vi "Handle Payload.vi"(8 "error in (no error)":errorcluster, 10 "Incoming Packets":u8[](array[numeric]) format="%08b", 11 "ControlPacket in":refnum<class "ControlPacket.lvclass">) -> (0 "error out":errorcluster, 1 "Payload Complete?":bool=TRUE, 2 "Remaining Packets":u8[](array[numeric]) format="%08b", 3 "ControlPacket out":refnum<class "ControlPacket.lvclass">)   [LabVIEW 2013, in "ControlPacket.lvclass"]
uses:
  ControlPacket.lvclass
  ControlPacket.lvclass/ControlPacket.ctl
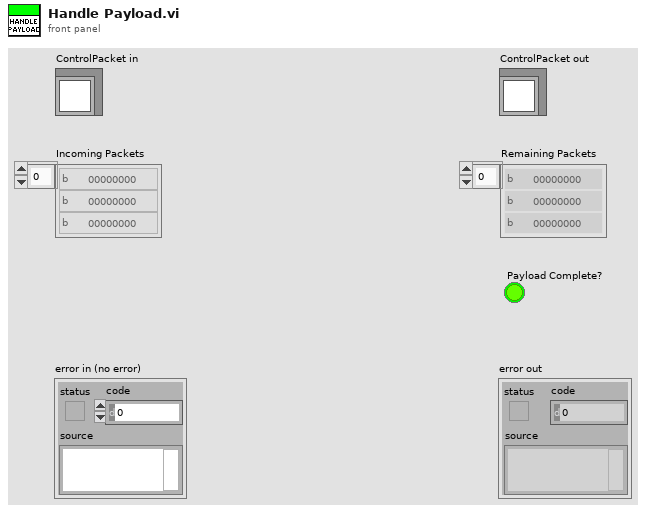
[diagram p1: front panel]
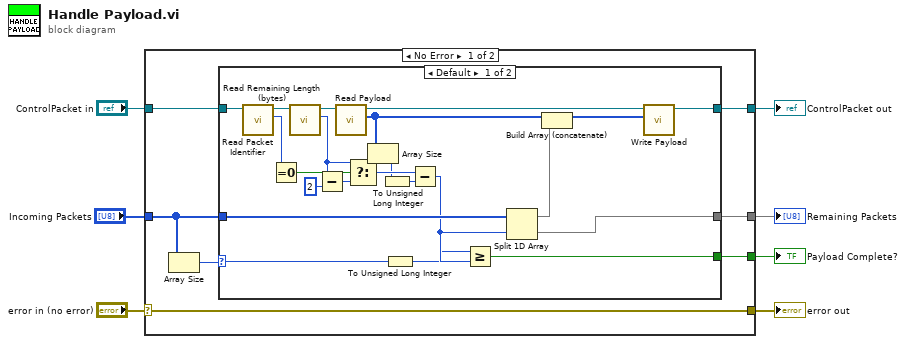
[diagram p0: block diagram]
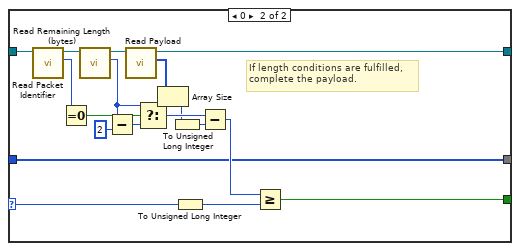
[diagram p2: hidden frame]
diagram:
  n1 = case shown="No Error" "error in (no error)" {
    selector: "error in (no error)" -> [w14 w57]
    tunnel: [w14 w57] -> w6
    tunnel: [w12 w56] -> w4
    tunnel: "ControlPacket in" -> [w13 w56]
    tunnel: "Incoming Packets" -> [w9 w55]
    tunnel: [w11 w55] -> w2
    tunnel: [w10 _] -> w1
    frame No Error {
      n2 = Array Size(array=w9) -> (size(s)=w8:i32)
      n3 = case shown="Default" w8 {
        selector: w8 -> [w17 w41]
        tunnel: w13 -> [w36 w54]
        tunnel: [w32 w38] -> w12
        tunnel: w9 -> [w23 w37]
        tunnel: [w20 w37] -> w11
        tunnel: [w15 w39] -> w10
        frame Default {
          n4 = call "Read Packet Identifier.vi"("ControlPacket in"=w36) -> ("Packet Identifier"=w31:u16, "ControlPacket out"=w35:refnum<class "ControlPacket.lvclass">)  [unwired: 9 in]
          n5 = Equal To 0?(x=w31) -> (x = 0?=w30:bool)
          n6 = call "Read Remaining Length (bytes).vi"("ControlPacket in"=w35) -> ("Remaining Length (bytes)"=w29:u32, "ControlPacket out"=w34:refnum<class "ControlPacket.lvclass">)  [unwired: 8 in, 1 out]
          n7 = Subtract(x=w29, y=u32 2) -> (x-y=w27:u32)
          n8 = call "Read Payload.vi"("ControlPacket in"=w34) -> ("Payload"=w22:u8[], "ControlPacket out"=w33:refnum<class "ControlPacket.lvclass">)  [unwired: 9 in]
          n9 = Select(t=w29, s=w30, f=w27) -> (s? t:f=w26:u32)
          n10 = Array Size(array=w22) -> (size(s)=w25:i32)
          n11 = To Unsigned Long Integer(number=w25) -> (unsigned 32bit integer=w24:u32)
          n12 = To Unsigned Long Integer(number=w17) -> (unsigned 32bit integer=w16:u32)
          n13 = Subtract(x=w26, y=w24) -> (x-y=w18:u32)
          n14 = Greater Or Equal?(x=w16, y=w18) -> (x >= y?=w15:bool)
          n15 = Split 1D Array(array=w23, index=w18) -> (first subarray=w21:u8[], second subarray=w20:u8[])
          n16 = Build Array (concatenate)(w22, w21) -> (w19:u8[])
          n17 = call "Write Payload.vi"("Payload"=w19, "ControlPacket in"=w33) -> ("ControlPacket out"=w32:refnum<class "ControlPacket.lvclass">)  [unwired: 9 in]
        }
        frame 0 {
          # "If length conditions are fulfilled,\ncomplete the payload."
          n18 = call "Read Packet Identifier.vi"("ControlPacket in"=w54) -> ("Packet Identifier"=w51:u16, "ControlPacket out"=w53:refnum<class "ControlPacket.lvclass">)  [unwired: 9 in]
          n19 = Equal To 0?(x=w51) -> (x = 0?=w50:bool)
          n20 = call "Read Remaining Length (bytes).vi"("ControlPacket in"=w53) -> ("Remaining Length (bytes)"=w49:u32, "ControlPacket out"=w52:refnum<class "ControlPacket.lvclass">)  [unwired: 8 in, 1 out]
          n21 = Subtract(x=w49, y=u32 2) -> (x-y=w47:u32)
          n22 = call "Read Payload.vi"("ControlPacket in"=w52) -> ("Payload"=w43:u8[], "ControlPacket out"=w38:refnum<class "ControlPacket.lvclass">)  [unwired: 9 in]
          n23 = Select(t=w49, s=w50, f=w47) -> (s? t:f=w46:u32)
          n24 = Array Size(array=w43) -> (size(s)=w45:i32)
          n25 = To Unsigned Long Integer(number=w45) -> (unsigned 32bit integer=w44:u32)
          n26 = To Unsigned Long Integer(number=w41) -> (unsigned 32bit integer=w40:u32)
          n27 = Subtract(x=w46, y=w44) -> (x-y=w42:u32)
          n28 = Greater Or Equal?(x=w42, y=w40) -> (x >= y?=w39:bool)
        }
      }
    }
    frame Error {
    }
  }
  "error out" <- w6
  "ControlPacket out" <- w4
  "Remaining Packets" <- w2
  "Payload Complete?" <- w1
